vi "sub_panel.vi"() -> ()   [LabVIEW 2024]
panel:
  out "Boolean":bool
  in  "knob":dbl(knob) scale=0.0..10.0
  out "numeric_test":dbl
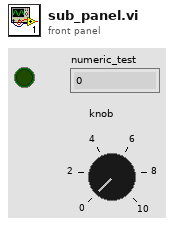
[diagram p1: front panel]
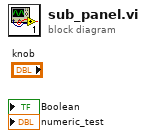
[diagram p0: block diagram]
diagram:
